vi "Get Process File Path from Settings Folder.vi"(11 "Settings Folder":path) -> (1 "Found?":bool, 3 "Process File Path":path)   [LabVIEW 2017, in "Test Executive Explorer.lvclass"]
uses:
  <vilib>/gpm_packages/@cs/Test-executive-builder/Example/Application/Test Executive Explorer/Test Executive Explorer/Test Executive Explorer.lvclass
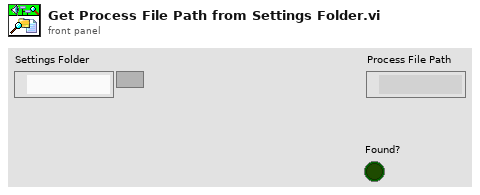
[diagram p1: front panel]
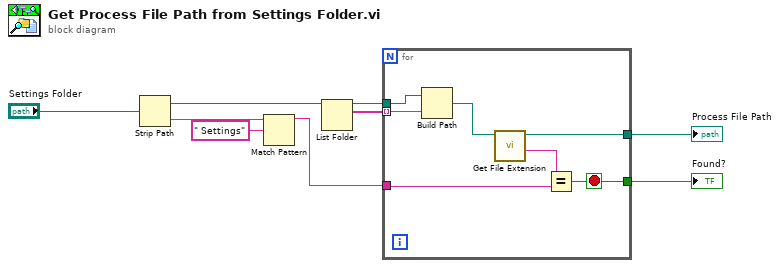
[diagram p0: block diagram]
diagram:
  n1 = Strip Path(path="Settings Folder") -> (stripped path=w8:path, name=w7:string)
  n2 = Match Pattern(string=w7, regular expression=" Settings") -> (before substring=w3:string)  [unwired: 1 in, 3 out]
  n3 = List Folder(path=w8) -> (path out=w4:path, filenames=w5:string[])  [unwired: 3 in, 2 out]
  n4 = for {
    tunnel: w5 -> [w16] mode=indexing
    tunnel: w4 -> [w15]
    tunnel: w3 -> [w13]
    tunnel: [w11] -> w2
    tunnel: [w10] -> w1
    stop <- w11 stop-if-true
    n5 = Build Path(base path=w15, name or relative path=w16) -> (appended path=w14:path)
    n6 = call <vilib>:"Get File Extension.vi"("file"=w14) -> ("filename without extension"=w12:string, "dup file"=w10:path)  [unwired: 6 in, 3 out]
    n7 = Equal?(x=w12, y=w13) -> (x = y?=w11:bool)
  }
  "Process File Path" <- w1
  "Found?" <- w2
